vi "oa_Check for Speed Profile Continuity.vi"(7 "reset in":bool, 8 "error in (no error)":errorcluster, 9 "speed profile":T1 {"speed [RPM]" format="%.2f"; "time [s]" format="%.2f"}) -> (0 "error out":errorcluster, 1 "speed profile dup":T1 {"speed [RPM]" format="%.2f"; "time [s]" format="%.2f"}, 5 "position not continuous":bool)   [LabVIEW 2017]
uses:
  <vilib>/addons/Sound and Vibration/Order Analysis/Tach Process/SubVIs/speed profile.ctl
  <vilib>/addons/Sound and Vibration/Order Analysis/Tach Process/SoundVib_TachProcess.lvlib
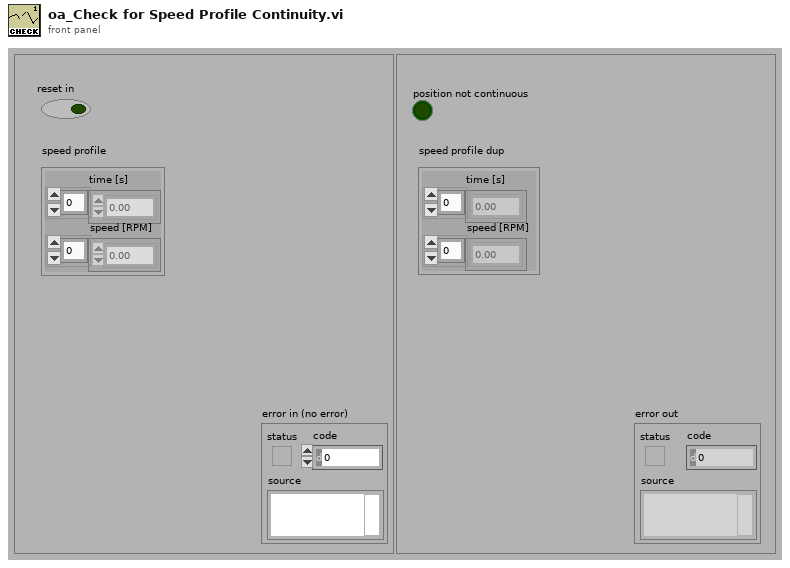
[diagram p1: front panel]
types:
  T1 = typedef "SoundVib_TachProcess.lvlib/speed profile.ctl" = cluster{"time [s]":dbl[], "speed [RPM]":dbl[]}
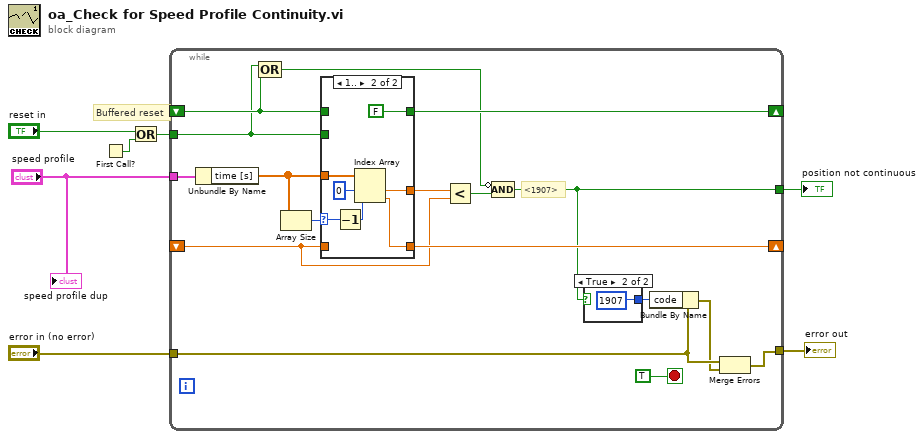
[diagram p0: block diagram]
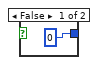
[diagram p2: hidden frame]
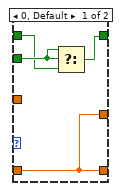
[diagram p3: hidden frame]
diagram:
  # "Buffered reset"
  n1 = First Call?() -> (First Call?: T/F=w6:bool)
  n2 = Or(x="reset in", y=w6) -> (x .or. y?=w4:bool)
  n3 = while {
    tunnel: "error in (no error)" -> [w11]
    shift-right: [w20] -> _
    shift-left: _ -> [w17]
    tunnel: "speed profile" -> [w23]
    shift-right: [w19] -> _
    shift-left: _ -> [w16]
    tunnel: w4 -> [w15]
    tunnel: [w9] -> w3
    tunnel: [w8] -> w2
    stop <- TRUE stop-if-true
    # "<1907>"
    n4 = Unbundle By Name(w23) -> ("time [s]"=w21:dbl[])
    n5 = Compound Arithmetic op=OR(w15, w16) -> (w13:bool)
    n6 = Array Size(array=w21) -> (size(s)=w22:i32)
    n7 = case shown="1.." w22 {
      selector: w22 -> [_ w35]
      tunnel: w21 -> [_ w37]
      tunnel: [w30 w33] -> w20
      tunnel: [w30 w32] -> w18
      tunnel: w17 -> [w30 _]
      tunnel: w15 -> [w29 _]
      tunnel: w16 -> [w28 _]
      tunnel: [w27 FALSE] -> w19
      frame 0, Default {
        n8 = Select(t=w29, s=w29, f=w28) -> (s? t:f=w27:bool)
      }
      frame 1.. {
        n9 = Decrement(x=w35) -> (x-1=w34:i32)
        n10 = Index Array(array=w37, index #1=0 ("index"), index #2=w34) -> (element #1=w32:dbl, element #2=w33:dbl)
      }
    }
    n11 = Less?(x=w18, y=w17) -> (x < y?=w14:bool)
    n12 = Compound Arithmetic op=AND(invert w13, w14) -> (w8:bool)
    n13 = case shown="True" w8 {
      tunnel: [0 ("code") 1907 ("code")] -> w12
      frame False {
      }
      frame True {
      }
    }
    n14 = Bundle By Name(cluster=w11, "code"=w12) -> (w10:errorcluster)
    n15 = Merge Errors(w11, w10) -> (w9:errorcluster)
  }
  "error out" <- w3
  "position not continuous" <- w2
  "speed profile dup" <- "speed profile"
